vi "Digital Reversed Order (I32).vi"(10 "radix":i32=2, 11 "X":i32[](array[numeric])) -> (0 "error":i32, 2 "Reversed Index":i32[](array[numeric]), 3 "Reversed {X}":i32[](array[numeric]))   [LabVIEW 2020, in "NI_AAL_SignalOperation.lvlib"]
doc: "Modifies the input array according to the digital-reversed order of the index."
uses:
  <vilib>/Analysis/NI_AAL_SignalOperation.lvlib
panel:
  # "Digital (n-based) Revered Order (I32)"
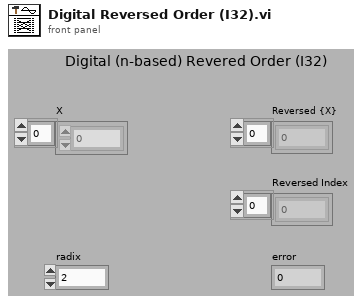
[diagram p1: front panel]
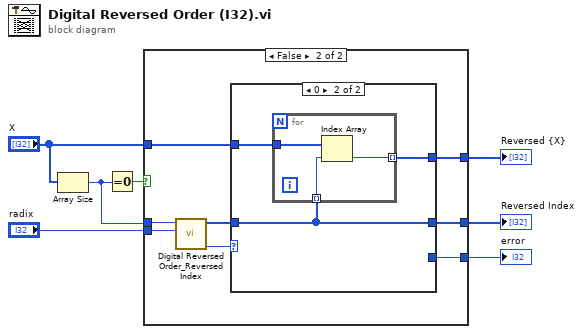
[diagram p0: block diagram]
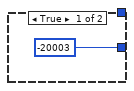
[diagram p2: hidden frame]
diagram:
  n1 = Array Size(array="X") -> (size(s)=w1:i32)
  n2 = Equal To 0?(x=w1) -> (x = 0?=w2:bool)
  n3 = case shown="False" w2 {
    tunnel: w1 -> [_ w16]
    tunnel: "X" -> [_ w13]
    tunnel: "radix" -> [_ w12]
    tunnel: [_ w11] -> w5
    tunnel: [_ w10] -> w4
    tunnel: [-20003 w9] -> w3
    frame True {
    }
    frame False {
      n4 = call <vilib>:"Digital Reversed Order_Reversed Index.vi"("radix"=w12, "length"=w16) -> ("error"=w14:i32, "Reversed Index"=w15:i32[])  [unwired: 8 in]
      n5 = case shown="0" w14 {
        selector: w14 -> [w17 _]
        tunnel: w15 -> [_ w18]
        tunnel: w13 -> [_ w20]
        tunnel: [_ w19] -> w11
        tunnel: [_ w18] -> w10
        tunnel: [w17 _] -> w9
        frame -1, Default {
        }
        frame 0 {
          n6 = for {
            tunnel: w20 -> [w23]
            tunnel: w18 -> [w22] mode=indexing
            tunnel: [w21] -> w19 mode=indexing
            n7 = Index Array(array=w23, index=w22) -> (element=w21:i32)
          }
        }
      }
    }
  }
  "Reversed {X}" <- w5
  "Reversed Index" <- w4
  "error" <- w3
